vi "LARelease.vi"(8 "Error Input":errorcluster, 11 "LiteAgent In":T1) -> (0 "Error Output":errorcluster)   [LabVIEW 2017, in "LiteAgentSDK.lvlib"]
uses:
  LiteAgentSDK.lvlib
  C:/Users/Jan/Projects/LiteAgentSDK-LabVIEW/Source/Bin/LiteAgentSDK.LabVIEW.dll
  Bin/LiteAgentSDK.LabVIEW.dll
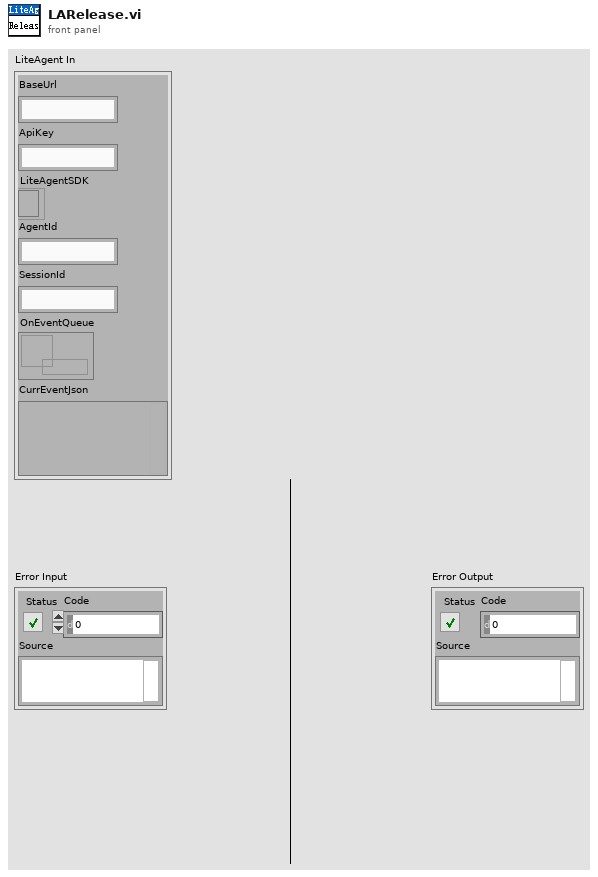
[diagram p1: front panel]
types:
  T1 = cluster{"BaseUrl":string, "ApiKey":string, "LiteAgentSDK":refnum<k24>, "AgentId":string, "SessionId":string, "OnEventQueue":refnum<queue>, "CurrEventJson":variant}
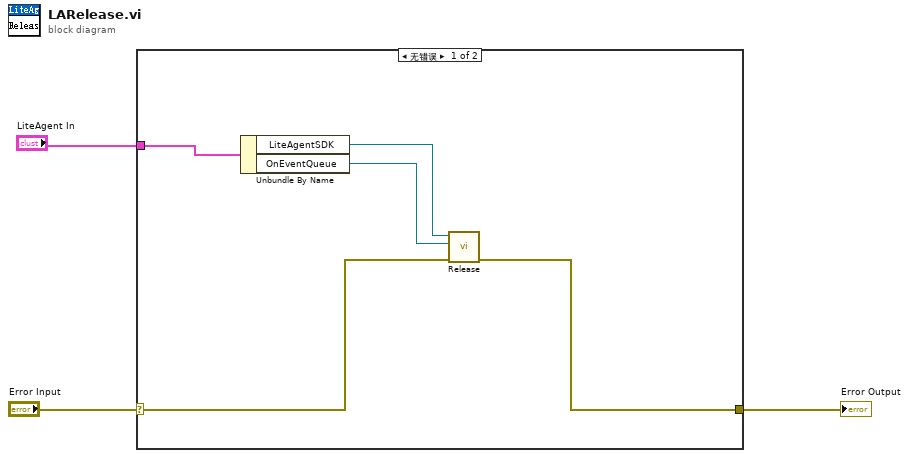
[diagram p0: block diagram]
diagram:
  n1 = case shown="无错误" "Error Input" {
    selector: "Error Input" -> [w8 w9]
    tunnel: [w7 w9] -> w2
    tunnel: "LiteAgent In" -> [w6 _]
    frame No Error {
      n2 = Unbundle By Name(w6) -> ("LiteAgentSDK"=w5:refnum<k24>, "OnEventQueue"=w4:refnum<queue>)
      n3 = call "Release.vi"("Error Input"=w8, "Queue In"=w4, "LiteAgentSDK Input"=w5) -> ("Error Output"=w7:errorcluster)  [unwired: 8 in]
    }
    frame Error {
    }
  }
  "Error Output" <- w2
